vi "判断括号中是否还有括号.vi"(1 "字符串":string) -> (0 "布尔":bool=TRUE)   [LabVIEW 2014]
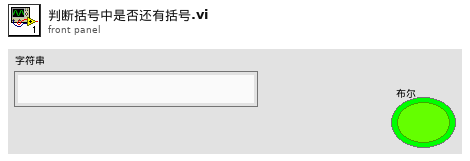
[diagram p1: front panel]
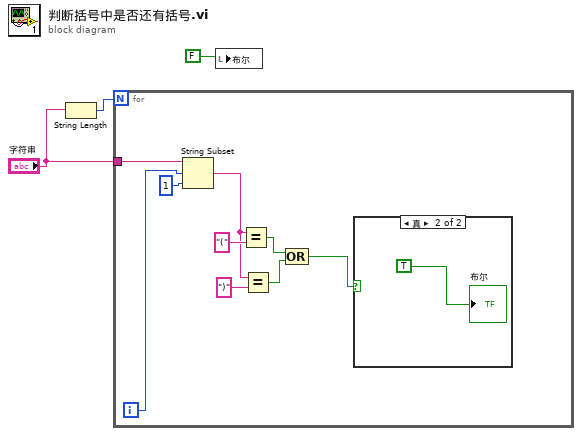
[diagram p0: block diagram]
diagram:
  n1 = String Length(string="字符串") -> (length=w2:i32)
  n2 = for {
    N: w2 -> [_]
    tunnel: "字符串" -> [w12]
    i -> [w5]
    n3 = String Subset(string=w12, offset (0)=w5, length (rest)=1 ("长度（剩余）")) -> (substring=w8:string)
    n4 = Equal?(x=w8, y="(") -> (x = y?=w7:bool)
    n5 = Equal?(x=w8, y=")") -> (x = y?=w6:bool)
    n6 = Compound Arithmetic op=OR(w7, w6) -> (w4:bool)
    n7 = case shown="真" w4 {
      frame False {
      }
      frame True {
        "布尔" <- TRUE
      }
    }
  }
  n8 = local write "布尔"(FALSE) -> ()
